vi "S30c_dll F95val.vi"(4 "error in":errorcluster, 5 "Target value [bar]":sgl, 6 "Comand":T1(ring), 7 "Dev Addr":u8=250) -> (0 "error out":errorcluster)   [LabVIEW 2014, in "K_S30c_dll.lvlib"]
uses:
  K_S30c_dll.lvlib
  s30c.dll
panel:
  # "Function 95val: Set Zero-point to Target value\n\nusing s30c.dll\nKeller AG für Druckmesstechnik, 29.5.08 b.v."
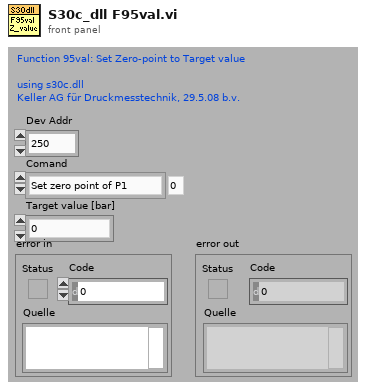
[diagram p1: front panel]
types:
  T1 = enum16{"Set zero point of P1", "Set default zero of P1", "Set zero point of P2", "Set defalut zero of P2", "not used", "not used_1", "Set zero point of CH0", "Set defalut zero of CH0"}
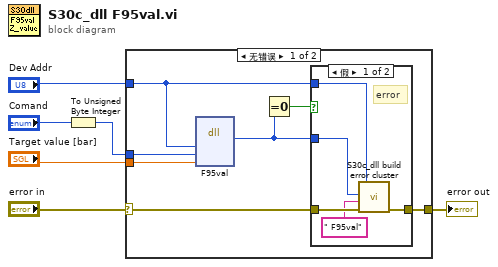
[diagram p0: block diagram]
diagram:
  n1 = To Unsigned Byte Integer(number="Comand") -> (unsigned 8bit integer=w2:u8)
  n2 = case shown="无错误" "error in" {
    selector: "error in" -> [w9 w20]
    tunnel: [w12 w20] -> w6
    tunnel: "Dev Addr" -> [w8 _]
    tunnel: w2 -> [w11 _]
    tunnel: "Target value [bar]" -> [w10 _]
    frame No Error {
      n3 = dll-call lib="PTH2Labs EworkSINOPEC北控自动相渗software2.08.5_dlls30c.dll" fn="F95val" label="dll call F95val"("DevAddr"=w8, "command"=w11, "sinVal"=w10) -> (w7:i16)  [unwired: 6 in, 2 out]
      n4 = Equal To 0?(x=w7) -> (x = 0?=w13:bool)
      n5 = case shown="假" w13 {
        tunnel: [w17 w19] -> w12
        tunnel: w9 -> [w18 w19]
        tunnel: w8 -> [w15 _]
        tunnel: w7 -> [w14 _]
        frame False {
          # "error"
          n6 = call "S30c_dll build error cluster.vi"("error in"=w18, "error Text"=" F95val", "error code"=w14, "Dev Addr"=w15) -> ("error out"=w17:errorcluster)  [unwired: 3 in]
        }
        frame True {
        }
      }
    }
    frame Error {
    }
  }
  "error out" <- w6
